vi "Bilan.vi"() -> ()   [LabVIEW 2024]
uses:
  <vilib>/Math Plots/3D Math Plots/3D Pie/3D Pie XCtrl/3D Pie.xctl
  <vilib>/Math Plots/3D Math Plots/3D Pie/3D Pie Datatype/Public/Plot Helper (Vector).vi
  <vilib>/Math Plots/3D Math Plots/3D Pie/3D Pie Datatype/3D Pie Datatype.lvclass
panel:
  out "new picture":picture
  in  "Historique":bool
  in  "Parametre":bool
  out "Horaire":string[](array[string])
  out "Immatricule":string[](array[string])
  out "Taux d'embouteillage":dbl(knob) scale=0.0..100.0
  out "Dernière Alerte de suspection":string
  out "Nombre de véhicules Total":refnum<class "3D Plot Datatype.lvclass">[](xcontrol)
  out "Nombre véhicules Suspects":string
  out "Nombre de véhicules Total":string
  in  "Regarder en direct":bool
  # "BILAN"
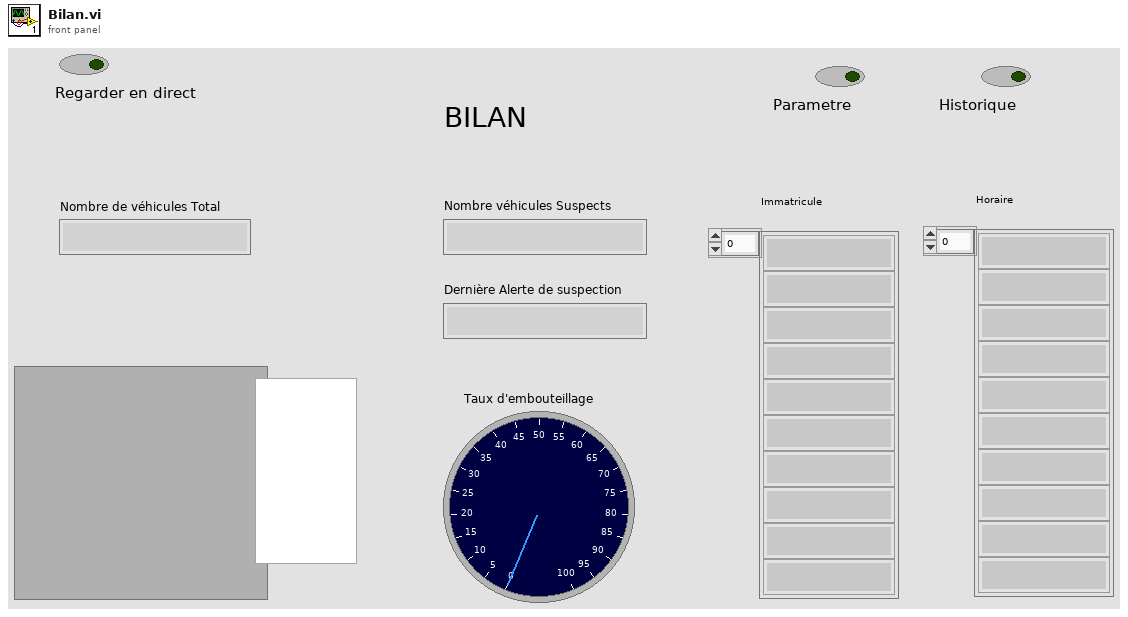
[diagram p1: front panel]
types:
  T1 = cluster{"Immatricule":string, "Color":u32, bool}[]
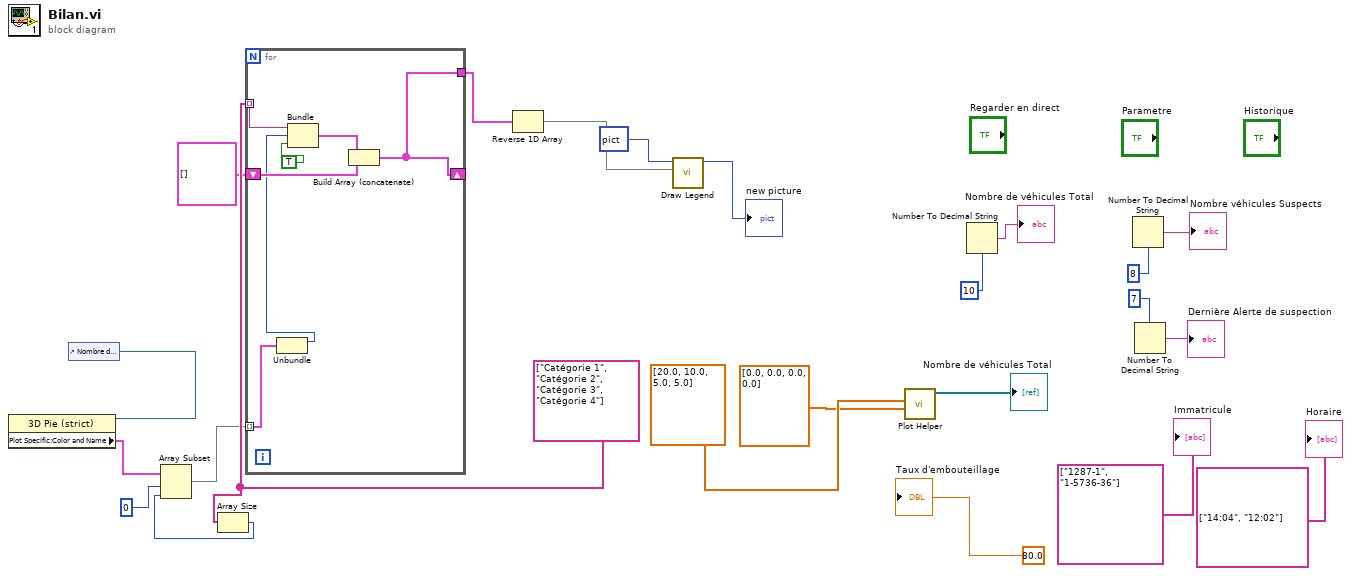
[diagram p0: block diagram]
diagram:
  w8 = string[] ["Catégorie 1", "Catégorie 2", "Catégorie 3", "Catégorie 4"] ("Immatricule")
  n1 = control-ref of="Nombre de véhicules Total"() -> (w11:refnum<vi>)
  n2 = property class="3D Pie (strict)"(reference=w11) -> ("Plot Specific:Color and Name"=w5:cluster{"Color":u32, "String":string}[])  [unwired: 1 in, 2 out]
  n3 = Array Size(array=w8) -> (size(s)=w7:i32)
  n4 = Array Subset(array=w5, index=0, length=w7) -> (w4:cluster{"Color":u32, "String":string}[])
  n5 = for {
    tunnel: w8 -> [w30] mode=indexing
    shift-right: [w27] -> _
    shift-left: T1 [] -> [w28]
    tunnel: [w27] -> w2
    tunnel: w4 -> [w24] mode=indexing
    n6 = Unbundle(w24) -> ("Color"=w25:u32)  [unwired: 1 out]
    n7 = Bundle("Immatricule"=w30, "Color"=w25, TRUE) -> (w29:cluster{"Immatricule":string, "Color":u32, bool})  [unwired: 1 in]
    n8 = Build Array (concatenate)(w29, w28) -> (w27:T1)
  }
  n9 = Reverse 1D Array(array=w2) -> (reversed array=w1:T1)
  n10 = call <vilib>:"Draw Legend.vi"("plot info"=w1, "picture"=picture data[5B]) -> ("new picture"=→"new picture":picture)  [unwired: 9 in]
  n11 = call-poly <vilib>:"Plot Helper.vi"("offset vector"=dbl[] [0.0, 0.0, 0.0, 0.0], "x vector"=dbl[] [20.0, 10.0, 5.0, 5.0]) -> ("3D Plot lvclass Array out"=→"Nombre de véhicules Total":refnum<class "3D Plot Datatype.lvclass">[])  [unwired: 1 in, 8 out]
  n12 = Number To Decimal String(number=10) -> (decimal integer string=→"Nombre de véhicules Total":string)  [unwired: 1 in]
  n13 = Number To Decimal String(number=8) -> (decimal integer string=→"Nombre véhicules Suspects":string)  [unwired: 1 in]
  n14 = Number To Decimal String(number=7) -> (decimal integer string=→"Dernière Alerte de suspection":string)  [unwired: 1 in]
  "Taux d'embouteillage" <- 80.0 ("Taux d'embouteillage")
  "Immatricule" <- string[] ["1287-1", "1-5736-36"] ("Immatricule")
  "Horaire" <- string[] ["14:04", "12:02"] ("Immatricule")
